vi "ParenthesisWrapper.vi"(11 "Input":string) -> (3 "Output":string)   [LabVIEW 2012]
uses:
  <vilib>/regexp/Match Regular Expression.xnode
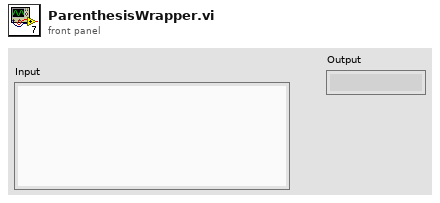
[diagram p1: front panel]
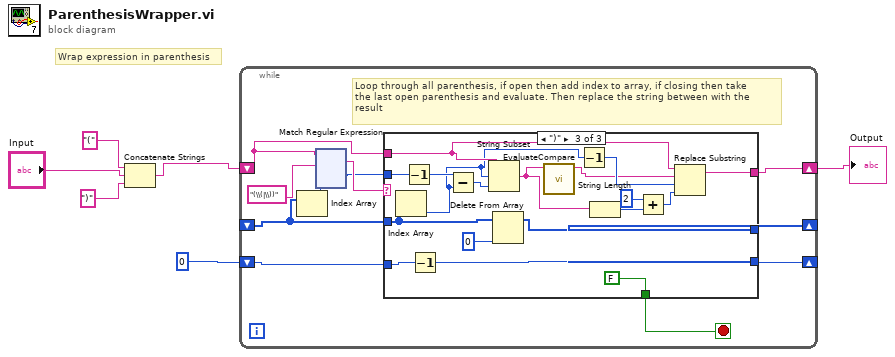
[diagram p0: block diagram]
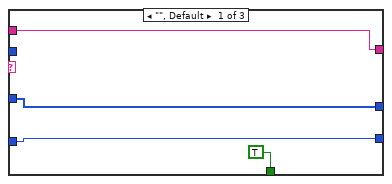
[diagram p2: hidden frame]
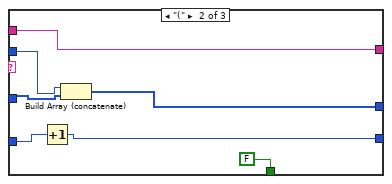
[diagram p3: hidden frame]
diagram:
  # "Wrap expression in parenthesis"
  n1 = Concatenate Strings("(", "Input", ")") -> (w3:string)
  n2 = while {
    shift-right: [w16] -> _
    shift-left: 0 -> [w17]
    shift-right: [w15] -> _
    shift-left: _ -> [w8]
    shift-right: [w14] -> w5
    shift-left: w3 -> [w12]
    stop <- w13 stop-if-true
    # "Loop through all parenthesis, if open then add index to array, if closing then take\nthe last open parenthesis and evaluate. Then replace the string between with the \nresult"
    n3 = Index Array(array=w8) -> (element=w7:i32)  [unwired: 1 in]
    n4 = xnode "Match Regular Expression"("input string"=w12, "regular expression"="(\\(|\\))", "offset (0)"=w7) -> ("whole match"=w10:string, "offset past match"=w9:i32)  [unwired: 3 in, 3 out]
    n5 = case shown="\")\"" w10 {
      tunnel: w17 -> [w132 w139 w157]
      tunnel: [w132 w138 w156] -> w16
      tunnel: w8 -> [w131 w133 w155]
      tunnel: [w131 w137 w154] -> w15
      tunnel: w9 -> [_ w134 w143]
      tunnel: w12 -> [w129 w135 w149]
      tunnel: [w129 w135 w148] -> w14
      tunnel: [TRUE FALSE FALSE] -> w13
      frame "", Default {
      }
      frame "(" {
        n6 = Increment(x=w139) -> (x+1=w138:i32)
        n7 = Build Array (concatenate)(w134, w133) -> (w137:i32[])
      }
      frame ")" {
        n8 = Index Array(array=w155) -> (element=w141:i32)  [unwired: 1 in]
        n9 = Decrement(x=w143) -> (x-1=w142:i32)
        n10 = Decrement(x=w157) -> (x-1=w156:i32)
        n11 = Subtract(x=w142, y=w141) -> (x-y=w153:i32)
        n12 = String Subset(string=w149, offset (0)=w141, length (rest)=w153) -> (substring=w150:string)
        n13 = Delete From Array(array=w155, index=0) -> (array with subset deleted=w154:i32[])  [unwired: 1 in, 1 out]
        n14 = call "EvaluateCompare.vi"("Input"=w150) -> ("Output"=w151:string)  [unwired: 9 in, 1 out]
        n15 = Decrement(x=w141) -> (x-1=w152:i32)
        n16 = String Length(string=w150) -> (length=w146:i32)
        n17 = Add(x=2, y=w146) -> (x+y=w144:i32)
        n18 = Replace Substring(2:w144, 3:w152, 4:w151, 5:w149) -> (1:w148:string)  [unwired: 1 out]
      }
    }
  }
  "Output" <- w5
